vi "M-686 Stage Engine.vi"(0 "Notifier Name":string, 11 "COM Port":string[](array[string])) -> ()   [LabVIEW 2016]
uses:
  Stages Controls/Stage Notifier Element.ctl
  Stages Controls/Stage Actions.ctl
  Stages Controls/Stage Status.ctl
  <vilib>/Instr/_visa.llb/VISA Configure Serial Port (Instr).vi
panel:
  in  "Quit":bool
  in  "Halt":bool
  in  "Home":bool
  in  "Get Position":bool
  in  "Y Position (µm)":dbl format="%#_4g"
  in  "X Position (µm)":dbl format="%#_4g"
  in  "XY Step Size (µm)":dbl format="%#_4g"
  in  "Up":bool
  in  "Down":bool
  in  "Left":bool
  in  "Right":bool
  in  "ReInitialize":bool
  in  "Error":bool
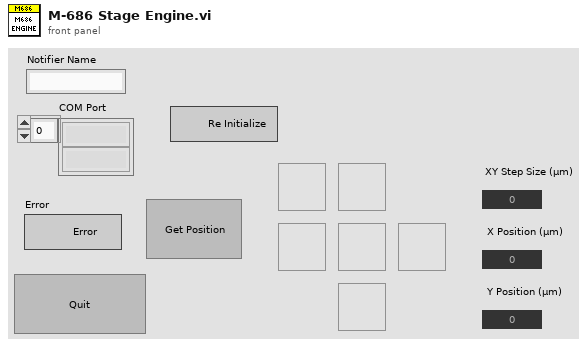
[diagram p1: front panel]
types:
  T1 = typedef "Stage Notifier Element.ctl" = cluster{"Action":T2, "Axis":bool[], "Setpoint":dbl[], "Velocity":dbl, "Cmd Recvd?":bool, "Position":dbl[], "Status":T3, "Misc":variant}
  T2 = typedef "Stage Actions.ctl" = enum16{"Get Position", "MVR", "MOVE", "HALT", "ONTARGET", "ERROR", "REFERENCE", "INIT", "VELOCITY", "STATUS", "EXIT", "HOME", "ZEROPOS", "NANOPOS", "ANALOG", "QUIT"}
  T3 = typedef "Stage Status.ctl" = enum16{"Error", "Abort", "Busy", "On Target"}
  T4 = enum32{"Invalid", "Standard", "Closed", "Hidden", "Minimized", "Maximized"}
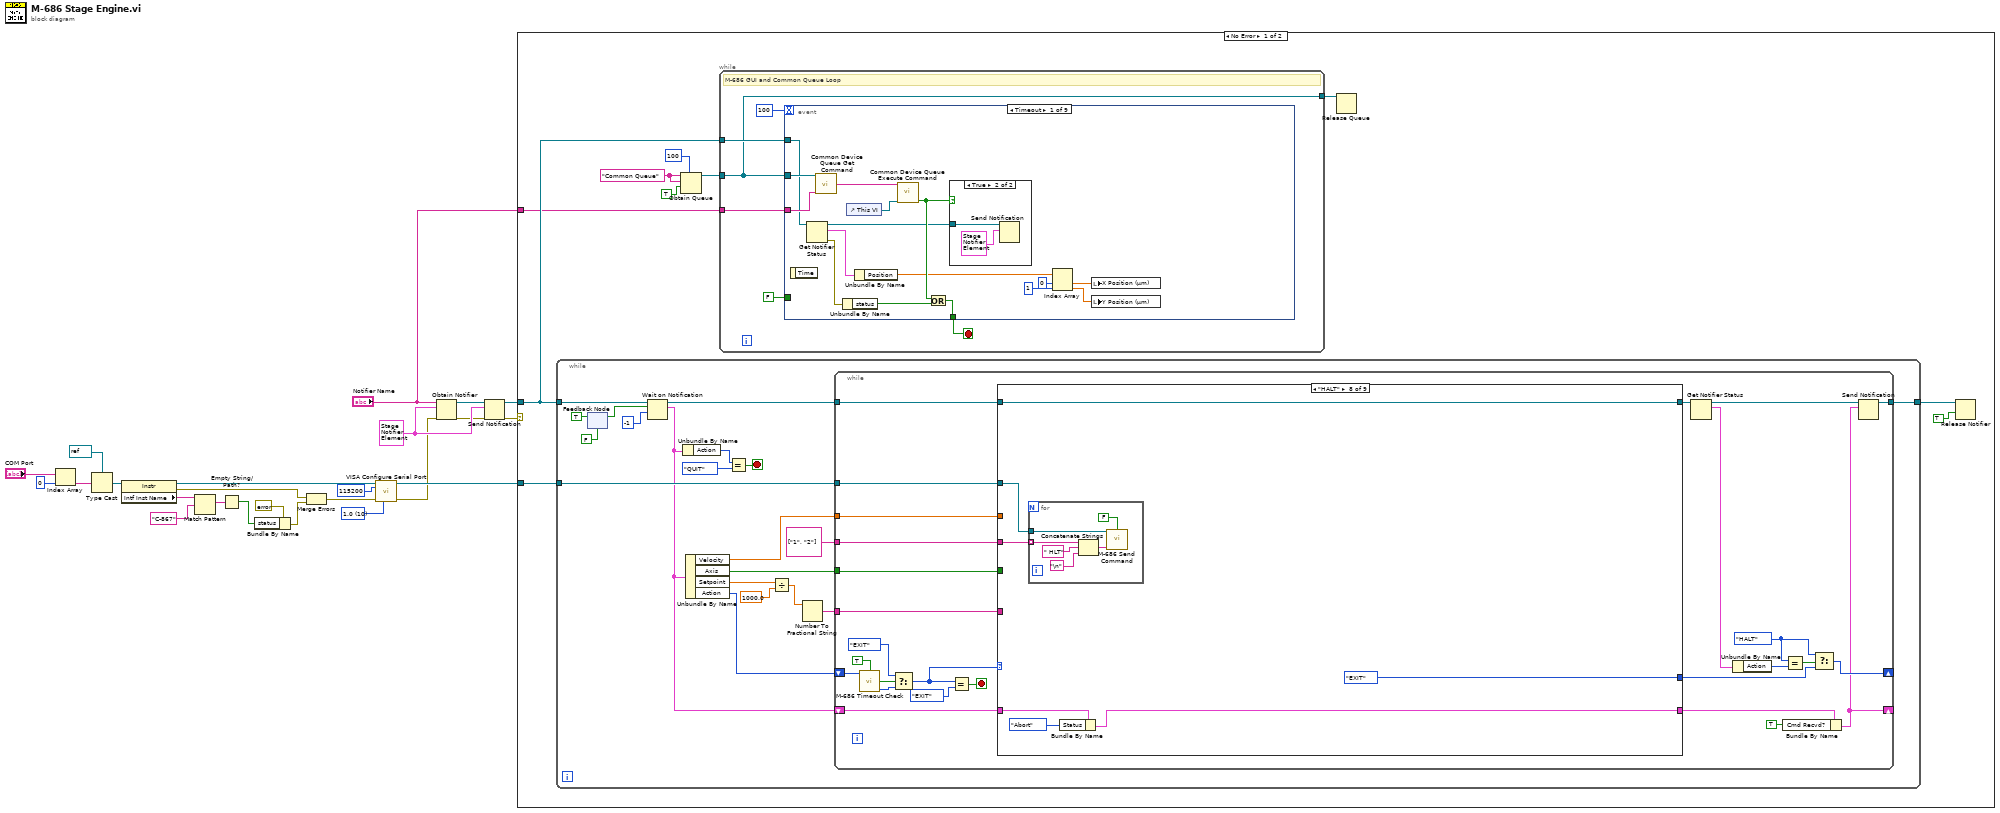
[diagram p0: block diagram]
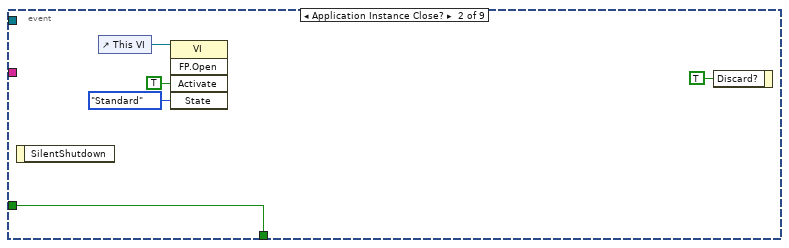
[diagram p3: hidden frame]
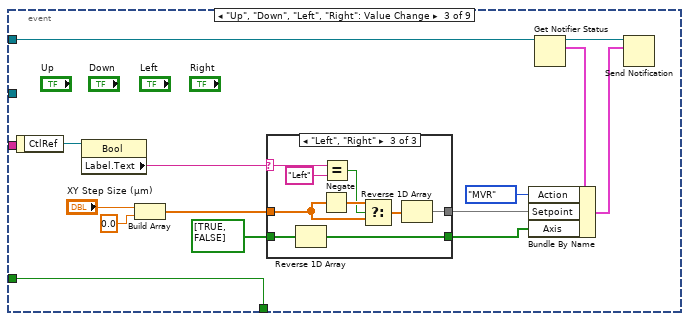
[diagram p4: hidden frame]
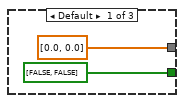
[diagram p5: hidden frame]
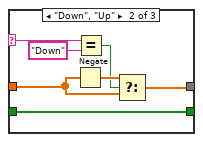
[diagram p6: hidden frame]
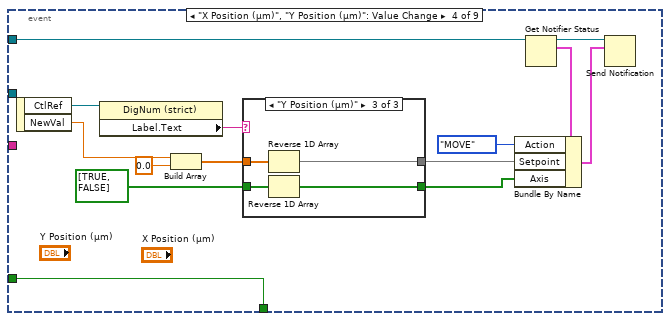
[diagram p7: hidden frame]
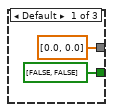
[diagram p8: hidden frame]
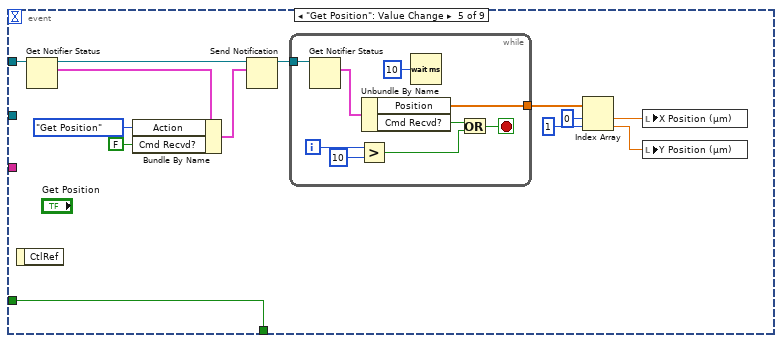
[diagram p10: hidden frame]
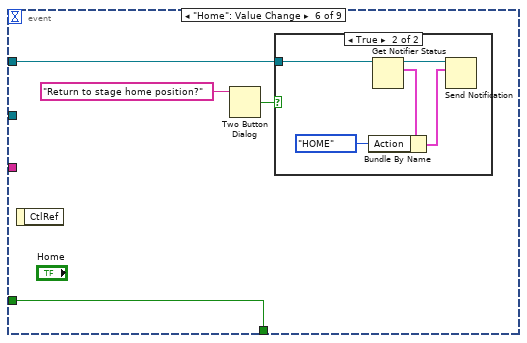
[diagram p11: hidden frame]
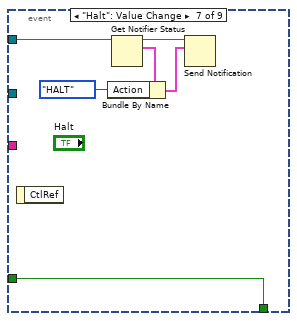
[diagram p13: hidden frame]
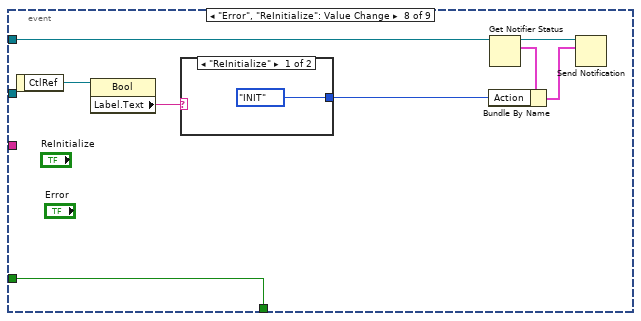
[diagram p14: hidden frame]
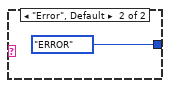
[diagram p15: hidden frame]
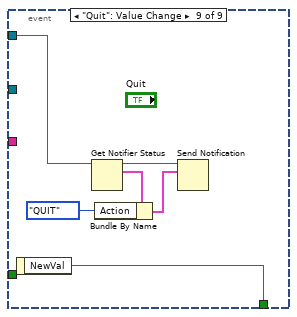
[diagram p16: hidden frame]
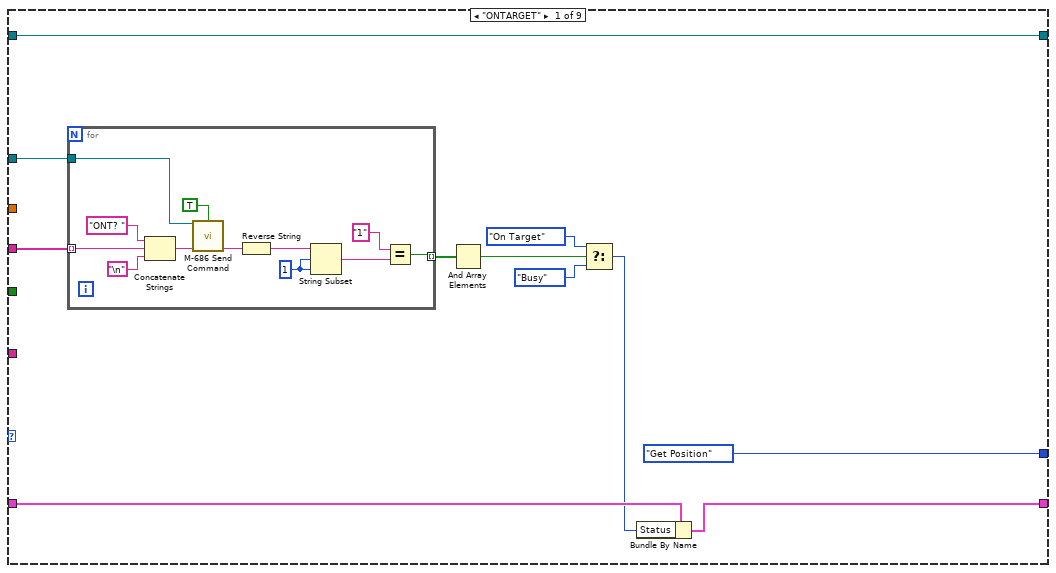
[diagram p17: hidden frame]
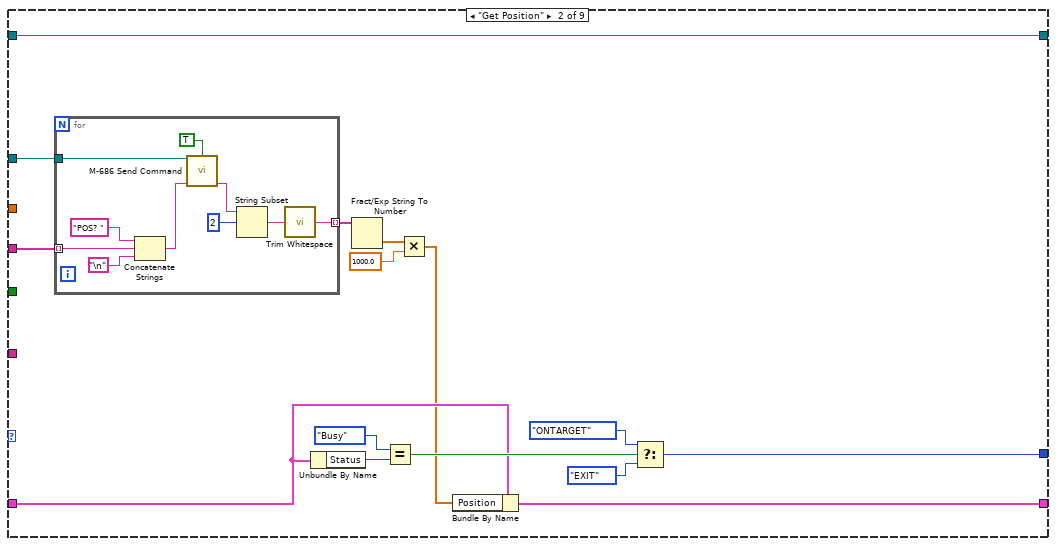
[diagram p18: hidden frame]
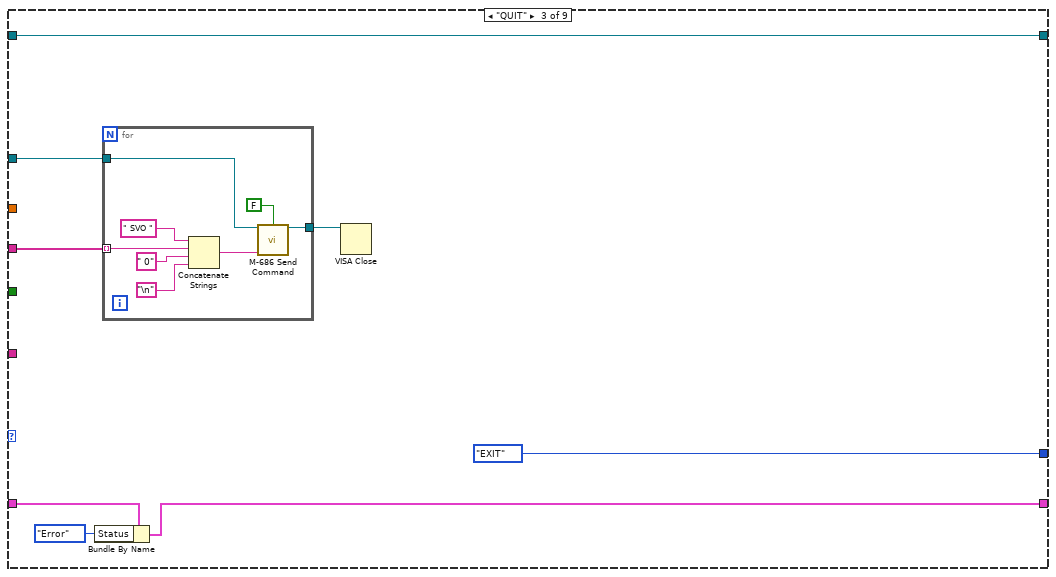
[diagram p19: hidden frame]
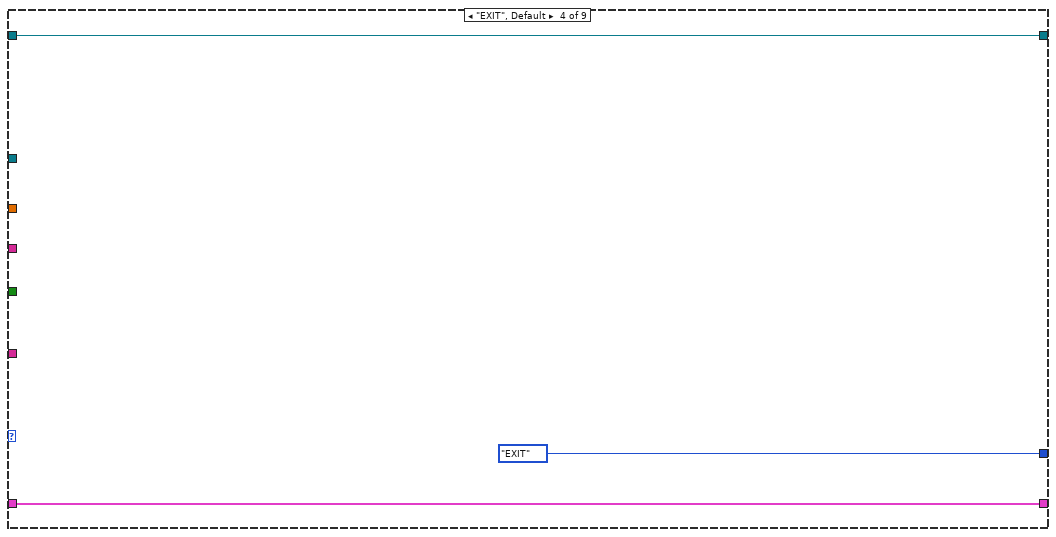
[diagram p20: hidden frame]
diagram:
  w6 = T1 {"Action"=enum."INIT", "Axis"=[], "Setpoint"=[], "Velocity"=0.5, "Cmd Recvd?"=FALSE, "Position"=[], "Status"=enum."Busy", "Misc"=variant} ("Stage Status")
  w11 = u16 10 items=["1.0"=10, "1.5"=15, "2.0"=20] ("stop bits (10: 1 bit)")
  n1 = Index Array(array="COM Port", index=0) -> (element=w17:string)
  n2 = Type Cast(type=refnum<visa-resource-name> refnum ("reference out"), x=w17) -> (*(type *) &x=w15:refnum<visa-resource-name>)
  n3 = property class="Instr"(reference=w15) -> (reference out=w10:refnum<visa-resource-name>, error out=w20:errorcluster, "Intf Inst Name"=w22:string)  [unwired: 1 in]
  n4 = Match Pattern(string=w22, regular expression="C-867") -> (match substring=w24:string)  [unwired: 1 in, 3 out]
  n5 = Empty String/Path?(string/path=w24) -> (empty?=w21:bool)
  n6 = Bundle By Name(cluster=errorcluster {"status"=FALSE, "code"=0, "source"=""} ("Error"), "status"=w21) -> (w19:errorcluster)
  n7 = Merge Errors(w20, w19) -> (w9:errorcluster)
  n8 = call-poly "VISA Configure Serial Port"("VISA resource name"=w10, "baud rate (9600)"=u32 115200, "error in (no error)"=w9, "stop bits (10: 1 bit)"=w11) -> ("VISA resource name out"=w8:refnum<visa-resource-name>, "error out"=w4:errorcluster)  [unwired: 10 in]
  n9 = Obtain Notifier(name (unnamed)="Notifier Name", notification data type=w6, error in (no error)=w4) -> (notifier out=w7:refnum<notifier>, error out=w5:errorcluster)  [unwired: 1 in, 1 out]
  n10 = Send Notification(notification=w6, notifier=w7, error in (no error)=w5) -> (notifier out=w3:refnum<notifier>, error out=w2:errorcluster)
  n11 = case shown="No Error" w2 {
    selector: w2 -> [_ w449]
    tunnel: w8 -> [w34 w450]
    tunnel: w3 -> [w27 w451]
    tunnel: "Notifier Name" -> [w26 _]
    frame No Error {
      w30 = "Common Queue" ("Unique Notifier Name")
      n12 = while {
        tunnel: w27 -> [w188]
        tunnel: w34 -> [w177]
        tunnel: [w174] -> w33
        stop <- w190 stop-if-true
        n13 = feedback-in #1(TRUE) -> ()
        n14 = feedback #1(FALSE) -> (w171:bool)
        n15 = Wait on Notification(notifier=w188, ignore previous (F)=w171, timeout in ms (-1)=-1) -> (notifier out=w176:refnum<notifier>, notification=w175:T1)  [unwired: 1 in, 2 out]
        n16 = Unbundle By Name(w175) -> ("Action"=w187:T2)
        n17 = Unbundle By Name(w175) -> ("Velocity"=w183:dbl, "Axis"=w182:bool[], "Setpoint"=w179:dbl[], "Action"=w181:T2)
        n18 = Equal?(x=w187, y=Stage_Actions."QUIT") -> (x = y?=w190:bool)
        n19 = Divide(x=w179, y=1000.0) -> (x/y=w180:dbl[])
        n20 = Number To Fractional String(number=w180) -> (F-format string=w184:string[])  [unwired: 3 in]
        n21 = while {
          tunnel: string[] ["1", "2"] -> [w217]
          shift-right: [w210] -> _
          shift-left: w181 -> [w207]
          tunnel: w182 -> [w214]
          tunnel: w183 -> [w213]
          tunnel: w184 -> [w215]
          shift-right: [w193] -> _
          shift-left: w175 -> [w212]
          tunnel: w177 -> [w216]
          tunnel: w176 -> [w192]
          tunnel: [w196] -> w174
          stop <- w208 stop-if-true
          w199 = Stage_Actions."HALT" ("Action")
          n22 = call "M-686 Timeout Check.vi"("Action"=w207, "User Input?"=TRUE) -> ("Timeout?"=w206:bool, "Action (Dup)"=w204:T2)  [unwired: 12 in]
          n23 = Select(t=Stage_Actions."EXIT" ("y"), s=w206, f=w204) -> (s? t:f=w203:T2)
          n24 = Equal?(x=w203, y=Stage_Actions."EXIT") -> (x = y?=w208:bool)
          n25 = case shown="\"HALT\"" w203 {
            selector: w203 -> [_ _ _ _ _ _ _ _ w407]
            tunnel: w217 -> [w226 w254 w272 _ _ w319 w358 w392 w419]
            tunnel: w216 -> [w228 w255 w273 _ w289 w310 w357 w387 w413]
            tunnel: w215 -> [_ _ _ _ _ _ _ _ w410]
            tunnel: w214 -> [_ _ _ _ _ _ _ _ w401]
            tunnel: w213 -> [_ _ _ _ _ _ _ _ w418]
            tunnel: [Stage_Actions."Get Position" ("Action") w252 Stage_Actions."EXIT" ("Action") Stage_Actions."EXIT" ("Action") w299 w318 w353 Stage_Actions."EXIT" ("Action") Stage_Actions."ONTARGET" ("Action")] -> w211
            tunnel: w212 -> [w221 w249 w270 w284 w297 w320 w351 w389 w415]
            tunnel: [w219 w247 w268 w284 w298 w321 w350 w388 w414] -> w195
            tunnel: w192 -> [w218 w241 w266 w282 w285 w305 w349 w386 w399]
            tunnel: [w218 w241 w266 w282 w285 w305 w349 w386 w399] -> w191
            frame "ONTARGET" {
              n26 = for {
                tunnel: [w238] -> w227 mode=indexing
                tunnel: w226 -> [w233] mode=indexing
                tunnel: w228 -> [w230]
                w234 = 1 ("length (rest)")
                n27 = Concatenate Strings("ONT? " ("string"), w233, "\n") -> (w232:string)
                n28 = call "M-686 Send Command.vi"("VISA Ref"=w230, "Wait for Reply?"=TRUE, "Command"=w232) -> ("Response"=w229:string)  [unwired: 10 in, 2 out]
                n29 = Reverse String(1:w229) -> (0:w235:string)
                n30 = String Subset(string=w235, offset (0)=w234, length (rest)=w234) -> (substring=w240:string)
                n31 = Equal?(x="1", y=w240) -> (x = y?=w238:bool)
              }
              n32 = And Array Elements(Boolean array=w227) -> (logical AND=w222:bool)
              n33 = Select(t=Stage_Status."On Target" ("Status"), s=w222, f=Stage_Status."Busy" ("Status")) -> (s? t:f=w220:T3)
              n34 = Bundle By Name(cluster=w221, "Status"=w220) -> (w219:T1)
            }
            frame "Get Position" {
              n35 = for {
                tunnel: [w265] -> w253 mode=indexing
                tunnel: w254 -> [w260] mode=indexing
                tunnel: w255 -> [w259]
                n36 = Concatenate Strings("POS? " ("string"), w260, "\n") -> (w258:string)
                n37 = call "M-686 Send Command.vi"("VISA Ref"=w259, "Wait for Reply?"=TRUE, "Command"=w258) -> ("Response"=w256:string)  [unwired: 10 in, 2 out]
                n38 = String Subset(string=w256, offset (0)=2) -> (substring=w261:string)  [unwired: 1 in]
                n39 = call <vilib>:"Trim Whitespace.vi"("string"=w261) -> ("trimmed string"=w265:string)  [unwired: 1 in]
              }
              n40 = Unbundle By Name(w249) -> ("Status"=w248:T3)
              n41 = Fract/Exp String To Number(string=w253) -> (number=w246:dbl[])  [unwired: 3 in, 1 out]
              n42 = Equal?(x=Stage_Status."Busy", y=w248) -> (x = y?=w250:bool)
              n43 = Multiply(x=w246, y=1000.0) -> (x*y=w243:dbl[])
              n44 = Bundle By Name(cluster=w249, "Position"=w243) -> (w247:T1)
              n45 = Select(t=Stage_Actions."ONTARGET" ("Action"), s=w250, f=Stage_Actions."EXIT" ("Action")) -> (s? t:f=w252:T2)
            }
            frame "QUIT" {
              n46 = Bundle By Name(cluster=w270, "Status"=Stage_Status."Error") -> (w268:T1)
              n47 = for {
                tunnel: w273 -> [w275]
                tunnel: w272 -> [w278] mode=indexing
                tunnel: [w274] -> w267
                n48 = Concatenate Strings(" SVO " ("string"), w278, " 0" ("string"), "\n") -> (w277:string)
                n49 = call "M-686 Send Command.vi"("VISA Ref"=w275, "Wait for Reply?"=FALSE, "Command"=w277) -> ("VISA Ref Out"=w274:refnum<visa-resource-name>)  [unwired: 10 in, 2 out]
              }
              n50 = VISA Close(VISA resource name=w267) -> ()  [unwired: 1 in, 1 out]
            }
            frame "EXIT", Default {
            }
            frame "ERROR" {
              n51 = Concatenate Strings(" ERR?" ("string"), "\n") -> (w287:string)
              n52 = call "M-686 Send Command.vi"("VISA Ref"=w289, "Wait for Reply?"=TRUE, "Command"=w287) -> ("Response"=w286:string)  [unwired: 10 in, 2 out]
              n53 = Reverse String(1:w286) -> (0:w294:string)
              n54 = String Subset(string=w294, offset (0)=1) -> (substring=w296:string)  [unwired: 1 in]
              n55 = Equal?(x=w296, y="0") -> (x = y?=w290:bool)
              n56 = Select(t=Stage_Status."Busy" ("Status"), s=w290, f=Stage_Status."Error" ("Status")) -> (s? t:f=w302:T3)
              n57 = Bundle By Name(cluster=w297, "Status"=w302) -> (w298:T1)
              n58 = Select(t=Stage_Actions."ONTARGET" ("Action"), s=w290, f=Stage_Actions."ERROR") -> (s? t:f=w299:T2)
            }
            frame "INIT" {
              n59 = Concatenate Strings(" ERR?" ("string"), "\n") -> (w307:string)
              n60 = Bundle By Name(cluster=w320, "Status"=Stage_Status."Busy") -> (w321:T1)
              n61 = call "M-686 Send Command.vi"("VISA Ref"=w310, "Wait for Reply?"=TRUE, "Command"=w307) -> ("VISA Ref Out"=w309:refnum<visa-resource-name>, "Response"=w306:string)  [unwired: 10 in, 1 out]
              n62 = Reverse String(1:w306) -> (0:w316:string)
              n63 = String Subset(string=w316, offset (0)=1) -> (substring=w314:string)  [unwired: 1 in]
              n64 = Equal?(x=w314, y="0") -> (x = y?=w311:bool)
              n65 = case shown="True" w311 {
                tunnel: w319 -> [_ w330]
                tunnel: [Stage_Actions."INIT" ("Action") w328] -> w318
                tunnel: w309 -> [_ w325]
                frame False {
                }
                frame True {
                  n66 = for {
                    tunnel: w330 -> [w344] mode=indexing
                    tunnel: w325 -> [w337]
                    tunnel: [w339] -> w324 mode=indexing
                    w343 = 1 ("length (rest)")
                    n67 = Concatenate Strings(" SVO " ("string"), w344, " 1" ("string"), "\n") -> (w336:string)
                    n68 = Concatenate Strings(" SVO? " ("string"), w344, "\n") -> (w333:string)
                    n69 = call "M-686 Send Command.vi"("VISA Ref"=w337, "Wait for Reply?"=FALSE, "Command"=w336) -> ("VISA Ref Out"=w334:refnum<visa-resource-name>)  [unwired: 10 in, 2 out]
                    n70 = call "M-686 Send Command.vi"("VISA Ref"=w334, "Wait for Reply?"=TRUE, "Command"=w333) -> ("Response"=w331:string)  [unwired: 10 in, 2 out]
                    n71 = Reverse String(1:w331) -> (0:w342:string)
                    n72 = String Subset(string=w342, offset (0)=w343, length (rest)=w343) -> (substring=w341:string)
                    n73 = Equal?(x=w341, y="1") -> (x = y?=w339:bool)
                  }
                  n74 = And Array Elements(Boolean array=w324) -> (logical AND=w326:bool)
                  n75 = Select(t=Stage_Actions."REFERENCE" ("Action"), s=w326, f=Stage_Actions."INIT" ("Action")) -> (s? t:f=w328:T2)
                }
              }
            }
            frame "REFERENCE" {
              n76 = for {
                tunnel: w358 -> [w383] mode=indexing
                tunnel: w357 -> [w377]
                tunnel: [w376] -> w354
                tunnel: [w378] -> w356 mode=indexing
                w381 = 1 ("length (rest)")
                n77 = Concatenate Strings(" FRF? " ("string"), w383, "\n") -> (w375:string)
                n78 = call "M-686 Send Command.vi"("VISA Ref"=w377, "Wait for Reply?"=TRUE, "Command"=w375) -> ("VISA Ref Out"=w376:refnum<visa-resource-name>, "Response"=w374:string)  [unwired: 10 in, 1 out]
                n79 = Reverse String(1:w374) -> (0:w382:string)
                n80 = String Subset(string=w382, offset (0)=w381, length (rest)=w381) -> (substring=w379:string)
                n81 = Equal?(x=w379, y="1") -> (x = y?=w378:bool)
              }
              n82 = Bundle By Name(cluster=w351, "Status"=Stage_Status."Busy") -> (w350:T1)
              n83 = And Array Elements(Boolean array=w356) -> (logical AND=w355:bool)
              n84 = case shown="False" w355 {
                tunnel: w354 -> [w360 _]
                tunnel: [w359 Stage_Actions."ONTARGET" ("Action")] -> w353
                frame False {
                  n85 = Two Button Dialog(message="M686", 1:"Skip" ("F button name (\"Cancel\")"), 2:"Reference" ("T button name (\"OK\")")) -> (T button?=w364:bool)
                  n86 = case shown="True" w364 {
                    tunnel: [Stage_Actions."HALT" ("Action") Stage_Actions."ONTARGET" ("Action")] -> w359
                    tunnel: w360 -> [_ w368]
                    frame False {
                    }
                    frame True {
                      n87 = Concatenate Strings("FRF" ("string"), "\n") -> (w367:string)
                      n88 = call "M-686 Send Command.vi"("VISA Ref"=w368, "Wait for Reply?"=FALSE, "Command"=w367) -> ()  [unwired: 10 in, 3 out]
                    }
                  }
                }
                frame True {
                }
              }
            }
            frame "HALT" {
              n89 = for {
                tunnel: w392 -> [w396] mode=indexing
                tunnel: w387 -> [w394]
                n90 = Concatenate Strings(w396, " HLT" ("string"), "\n") -> (w395:string)
                n91 = call "M-686 Send Command.vi"("VISA Ref"=w394, "Wait for Reply?"=FALSE, "Command"=w395) -> ()  [unwired: 10 in, 3 out]
              }
              n92 = Bundle By Name(cluster=w389, "Status"=Stage_Status."Abort") -> (w388:T1)
            }
            frame "MVR", "MOVE", "HOME" {
              n93 = Bundle By Name(cluster=w415, "Status"=Stage_Status."Busy") -> (w414:T1)
              n94 = Equal?(x=Stage_Actions."MVR", y=w407) -> (x = y?=w400:bool)
              n95 = Equal?(x=w407, y=Stage_Actions."HOME") -> (x = y?=w411:bool)
              n96 = Not(x=w411) -> (.not. x?=w406:bool)
              n97 = Select(t="MVR ", s=w400, f="MOV ") -> (s? t:f=w402:string)
              n98 = Select(t=w410, s=w406, f=string[] ["12.5", "12.5"]) -> (s? t:f=w409:string[])
              n99 = for {
                tunnel: w419 -> [w425] mode=indexing
                tunnel: w409 -> [w424] mode=indexing
                tunnel: w401 -> [w423] mode=indexing
                tunnel: w418 -> [w422]
                tunnel: w413 -> [w421]
                tunnel: w402 -> [w420]
                n100 = case shown="True" w423 {
                  tunnel: w425 -> [_ w433]
                  tunnel: w424 -> [_ w434]
                  tunnel: w421 -> [_ w427]
                  tunnel: w422 -> [_ w432]
                  tunnel: w420 -> [_ w426]
                  frame False {
                  }
                  frame True {
                    n101 = Equal To 0?(x=w432) -> (x = 0?=w431:bool)
                    n102 = call <vilib>:"Space Constant.vi"() -> ("String"=w435:string)
                    n103 = case shown="False" w431 {
                      tunnel: w433 -> [w443 _]
                      tunnel: w432 -> [w440 _]
                      tunnel: [w442 ""] -> w430
                      frame False {
                        n104 = Number To Fractional String(number=w440) -> (F-format string=w441:string)  [unwired: 3 in]
                        n105 = call <vilib>:"Space Constant.vi"() -> ("String"=w446:string)
                        n106 = Concatenate Strings("VEL ", w443, w446, w441, "\n") -> (w442:string)
                      }
                      frame True {
                      }
                    }
                    n107 = Concatenate Strings(w426, w433, w435, w434, "\n") -> (w429:string)
                    n108 = Build Array(w430, w429) -> (w428:string[])
                    n109 = for {
                      tunnel: w428 -> [w439] mode=indexing
                      tunnel: w427 -> [w437]
                      n110 = call "M-686 Send Command.vi"("VISA Ref"=w437, "Wait for Reply?"=FALSE, "Command"=w439) -> ()  [unwired: 10 in, 3 out]
                    }
                  }
                }
              }
            }
          }
          n111 = Get Notifier Status(notifier=w191) -> (notifier out=w197:refnum<notifier>, current notification=w198:T1)  [unwired: 1 in, 3 out]
          n112 = Unbundle By Name(w198) -> ("Action"=w200:T2)
          n113 = Bundle By Name(cluster=w195, "Cmd Recvd?"=TRUE) -> (w193:T1)
          n114 = Equal?(x=w199, y=w200) -> (x = y?=w201:bool)
          n115 = Select(t=w199, s=w201, f=w211) -> (s? t:f=w210:T2)
          n116 = Send Notification(notification=w193, notifier=w197) -> (notifier out=w196:refnum<notifier>)  [unwired: 1 in, 1 out]
        }
      }
      n117 = Obtain Queue(max queue size (-1, unlimited)=100, name (unnamed)=w30, element data type=w30, create if not found? (T)=TRUE) -> (queue out=w31:refnum<queue>)  [unwired: 1 in, 2 out]
      n118 = while {
        tunnel: w31 -> [w35]
        tunnel: w26 -> [w38]
        tunnel: w27 -> [w39]
        tunnel: [w35] -> w25
        stop <- w37 stop-if-true
        # "M-686 GUI and Common Queue Loop"
        n119 = event shown="[0] Timeout" {
          selector: _ -> [_ _ _ _ _ _ _ _ _]
          dyn-events: _ -> [_ _ _ _ _ _ _ _ _]
          timeout: 100 -> [_ _ _ _ _ _ _ _ _]
          tunnel: w35 -> [w50 _ _ _ _ _ _ _ _]
          tunnel: w39 -> [w47 _ w70 w102 w129 w140 w153 w159 w170]
          tunnel: w38 -> [w49 _ _ _ _ _ _ _ _]
          tunnel: [w48 w63 w73 w109 w130 w142 w154 w162 w166] -> w37
          tunnel: FALSE -> [_ w63 w73 w109 w130 w142 w154 w162 _]
          event Timeout {
            n120 = event-data() -> ()  [unwired: 1 in, 1 out]
            n121 = Get Notifier Status(notifier=w47) -> (notifier out=w51:refnum<notifier>, current notification=w46:T1, error out=w56:errorcluster)  [unwired: 1 in, 2 out]
            n122 = call "Common Device Queue Get Command.vi"("Common Queue"=w50, "Notifier Name"=w49) -> ("Command"=w55:string)  [unwired: 12 in, 1 out]
            n123 = Unbundle By Name(w56) -> ("status"=w53:bool)
            n124 = control-ref of="This VI"() -> (w54:refnum<vi>)
            n125 = Unbundle By Name(w46) -> ("Position"=w41:dbl[])
            n126 = call "Common Device Queue Execute Command.vi"("Common Command"=w55, "VI Refnum"=w54) -> ("Quit?"=w52:bool)  [unwired: 12 in, 1 out]
            n127 = Or(x=w52, y=w53) -> (x .or. y?=w48:bool)
            n128 = case shown="True" w52 {
              tunnel: w51 -> [_ w58]
              frame False {
              }
              frame True {
                n129 = Send Notification(notification=T1 {"Action"=enum."QUIT", "Axis"=[], "Setpoint"=[], "Velocity"=0.5, "Cmd Recvd?"=FALSE, "Position"=[], "Status"=enum."Error", "Misc"=variant} ("Stage Status"), notifier=w58) -> ()  [unwired: 1 in, 2 out]
              }
            }
            n130 = Index Array(array=w41, index #1=0 ("index"), index #2=1 ("index")) -> (element #1=w45:dbl, element #2=w44:dbl)
            n131 = local write "X Position (µm)"(w45) -> ()
            n132 = local write "Y Position (µm)"(w44) -> ()
          }
          event Application Instance Close? {
            n133 = event-data() -> ()  [unwired: 1 in, 1 out]
            n134 = control-ref of="This VI"() -> (w60:refnum<vi>)
            n135 = invoke class="VI" method="FP.Open"(reference=w60, "Activate"=TRUE ("Activate?"), "State"=T4."Standard") -> ()  [unwired: 2 in, 5 out]
            n136 = event-data("Discard?"=TRUE) -> ()  [unwired: 1 in, 1 out]
          }
          event "Up", "Down", "Left", "Right": Value Change {
            n137 = event-data() -> ("CtlRef"=w72:refnum<vi>)  [unwired: 1 in]
            n138 = property class="Bool"(reference=w72) -> ("Label.Text"=w77:string)  [unwired: 1 in, 2 out]
            n139 = Build Array("XY Step Size (µm)", 0.0 ("element")) -> (w75:dbl[])
            n140 = case shown="\"Left\", \"Right\"" w77 {
              selector: w77 -> [_ w86 w92]
              tunnel: w75 -> [_ w83 w91]
              tunnel: bool[] [TRUE, FALSE] -> [_ w80 w89]
              tunnel: [dbl[] [0.0, 0.0] w82 w88] -> w68
              tunnel: [bool[] [FALSE, FALSE] w80 w87] -> w67
              frame Default {
              }
              frame "Down", "Up" {
                n141 = Negate(x=w83) -> (-x=w84:dbl[])
                n142 = Equal?(x=w86, y="Down") -> (x = y?=w81:bool)
                n143 = Select(t=w84, s=w81, f=w83) -> (s? t:f=w82:dbl[])
              }
              frame "Left", "Right" {
                n144 = Reverse 1D Array(array=w89) -> (reversed array=w87:bool[])
                n145 = Negate(x=w91) -> (-x=w94:dbl[])
                n146 = Equal?(x=w92, y="Left") -> (x = y?=w93:bool)
                n147 = Select(t=w94, s=w93, f=w91) -> (s? t:f=w90:dbl[])
                n148 = Reverse 1D Array(array=w90) -> (reversed array=w88:dbl[])
              }
            }
            n149 = Get Notifier Status(notifier=w70) -> (notifier out=w65:refnum<notifier>, current notification=w69:T1)  [unwired: 1 in, 3 out]
            n150 = Bundle By Name(cluster=w69, "Action"=Stage_Actions."MVR", "Setpoint"=w68, "Axis"=w67) -> (w64:T1)
            n151 = Send Notification(notification=w64, notifier=w65) -> ()  [unwired: 1 in, 2 out]
          }
          event "X Position (µm)", "Y Position (µm)": Value Change {
            n152 = event-data() -> ("CtlRef"=w104:refnum<vi>, "NewVal"=w103:dbl)  [unwired: 1 in]
            n153 = property class="DigNum (strict)"(reference=w104) -> ("Label.Text"=w107:string)  [unwired: 1 in, 2 out]
            n154 = Build Array(w103, 0.0 ("element")) -> (w108:dbl[])
            n155 = case shown="\"Y Position (µm)\"" w107 {
              tunnel: w108 -> [_ w113 w117]
              tunnel: bool[] [TRUE, FALSE] -> [_ w112 w116]
              tunnel: [dbl[] [0.0, 0.0] w113 w115] -> w99
              tunnel: [bool[] [FALSE, FALSE] w112 w114] -> w98
              frame Default {
              }
              frame "X Position (µm)" {
              }
              frame "Y Position (µm)" {
                n156 = Reverse 1D Array(array=w117) -> (reversed array=w115:dbl[])
                n157 = Reverse 1D Array(array=w116) -> (reversed array=w114:bool[])
              }
            }
            n158 = Get Notifier Status(notifier=w102) -> (notifier out=w101:refnum<notifier>, current notification=w100:T1)  [unwired: 1 in, 3 out]
            n159 = Bundle By Name(cluster=w100, "Action"=Stage_Actions."MOVE", "Setpoint"=w99, "Axis"=w98) -> (w96:T1)
            n160 = Send Notification(notification=w96, notifier=w101) -> ()  [unwired: 1 in, 2 out]
          }
          event "Get Position": Value Change {
            n161 = event-data() -> ()  [unwired: 1 in, 1 out]
            n162 = Get Notifier Status(notifier=w129) -> (notifier out=w128:refnum<notifier>, current notification=w127:T1)  [unwired: 1 in, 3 out]
            n163 = Bundle By Name(cluster=w127, "Action"=Stage_Actions."Get Position", "Cmd Recvd?"=FALSE) -> (w124:T1)
            n164 = Send Notification(notification=w124, notifier=w128) -> (notifier out=w123:refnum<notifier>)  [unwired: 1 in, 1 out]
            n165 = while {
              tunnel: w123 -> [w139]
              tunnel: [w131] -> w122
              i -> [w135]
              stop <- w132 stop-if-true
              n166 = Get Notifier Status(notifier=w139) -> (current notification=w138:T1)  [unwired: 1 in, 4 out]
              n167 = Greater?(x=w135, y=10) -> (0:w133:bool)
              n168 = Unbundle By Name(w138) -> ("Position"=w131:dbl[], "Cmd Recvd?"=w134:bool)
              n169 = Wait (ms)(milliseconds to wait=u32 10) -> ()  [unwired: 1 out]
              n170 = Or(x=w134, y=w133) -> (x .or. y?=w132:bool)
            }
            n171 = Index Array(array=w122, index #1=0 ("index"), index #2=1 ("index")) -> (element #1=w119:dbl, element #2=w118:dbl)
            n172 = local write "X Position (µm)"(w119) -> ()
            n173 = local write "Y Position (µm)"(w118) -> ()
          }
          event "Home": Value Change {
            n174 = event-data() -> ()  [unwired: 1 in, 1 out]
            n175 = Two Button Dialog(message="Return to stage home position?") -> (T button?=w141:bool)  [unwired: 2 in]
            n176 = case shown="True" w141 {
              tunnel: w140 -> [_ w148]
              frame False {
              }
              frame True {
                n177 = Get Notifier Status(notifier=w148) -> (notifier out=w147:refnum<notifier>, current notification=w146:T1)  [unwired: 1 in, 3 out]
                n178 = Bundle By Name(cluster=w146, "Action"=Stage_Actions."HOME") -> (w145:T1)
                n179 = Send Notification(notification=w145, notifier=w147) -> ()  [unwired: 1 in, 2 out]
              }
            }
          }
          event "Halt": Value Change {
            n180 = event-data() -> ()  [unwired: 1 in, 1 out]
            n181 = Get Notifier Status(notifier=w153) -> (notifier out=w152:refnum<notifier>, current notification=w151:T1)  [unwired: 1 in, 3 out]
            n182 = Bundle By Name(cluster=w151, "Action"=Stage_Actions."HALT") -> (w150:T1)
            n183 = Send Notification(notification=w150, notifier=w152) -> ()  [unwired: 1 in, 2 out]
          }
          event "Error", "ReInitialize": Value Change {
            n184 = event-data() -> ("CtlRef"=w161:refnum<vi>)  [unwired: 1 in]
            n185 = property class="Bool"(reference=w161) -> ("Label.Text"=w160:string)  [unwired: 1 in, 2 out]
            n186 = case shown="\"ReInitialize\"" w160 {
              tunnel: [Stage_Actions."INIT" ("Action") Stage_Actions."ERROR" ("Action")] -> w155
              frame "ReInitialize" {
              }
              frame "Error", Default {
              }
            }
            n187 = Get Notifier Status(notifier=w159) -> (notifier out=w158:refnum<notifier>, current notification=w157:T1)  [unwired: 1 in, 3 out]
            n188 = Bundle By Name(cluster=w157, "Action"=w155) -> (w156:T1)
            n189 = Send Notification(notification=w156, notifier=w158) -> ()  [unwired: 1 in, 2 out]
          }
          event "Quit": Value Change {
            n190 = event-data() -> ("NewVal"=w166:bool)  [unwired: 1 in]
            n191 = Get Notifier Status(notifier=w170) -> (notifier out=w169:refnum<notifier>, current notification=w168:T1)  [unwired: 1 in, 3 out]
            n192 = Bundle By Name(cluster=w168, "Action"=Stage_Actions."QUIT") -> (w167:T1)
            n193 = Send Notification(notification=w167, notifier=w169) -> ()  [unwired: 1 in, 2 out]
          }
        }
      }
      n194 = Release Queue(queue=w25) -> ()  [unwired: 2 in, 3 out]
      n195 = Release Notifier(notifier=w33, force destroy? (F)=TRUE) -> ()  [unwired: 1 in, 3 out]
    }
    frame Error {
      n196 = VISA Close(VISA resource name=w450, error in (no error)=w449) -> (error out=w448:errorcluster)
      n197 = Release Notifier(notifier=w451, force destroy? (F)=TRUE, error in (no error)=w448) -> (error out=w456:errorcluster)  [unwired: 2 out]
      n198 = Unbundle By Name(w456) -> ("source"=w453:string)
      n199 = Concatenate Strings("M-686 (XY Sample Stage) Initialization Error", "\r", w453) -> (w452:string)
      n200 = One Button Dialog(message=w452) -> ()  [unwired: 1 in, 1 out]
    }
  }
